vi "Visualize_MutationHistory_Path.vi"(8 "error in (no error)":errorcluster, 10 "LVClass library Path":path, 11 "class reference":refnum<vi>) -> (0 "error out":errorcluster)   [LabVIEW 2019, in "BlueSerializationScripts.lvlib"]
uses:
  BlueSerializationScripts.lvlib
  BlueUtilityScripts/BlueUtilityScripts.lvlib
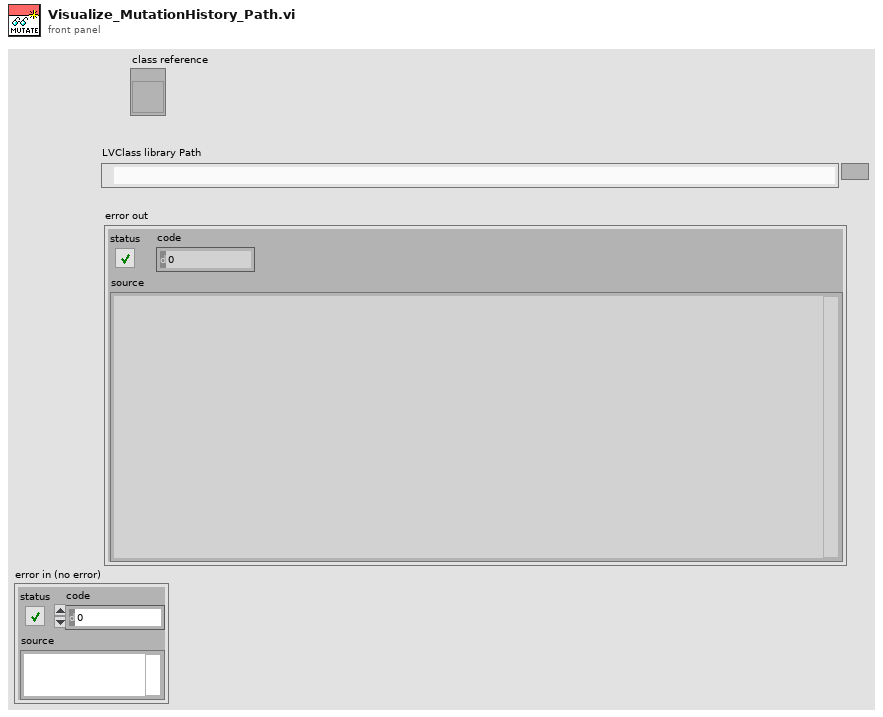
[diagram p1: front panel]
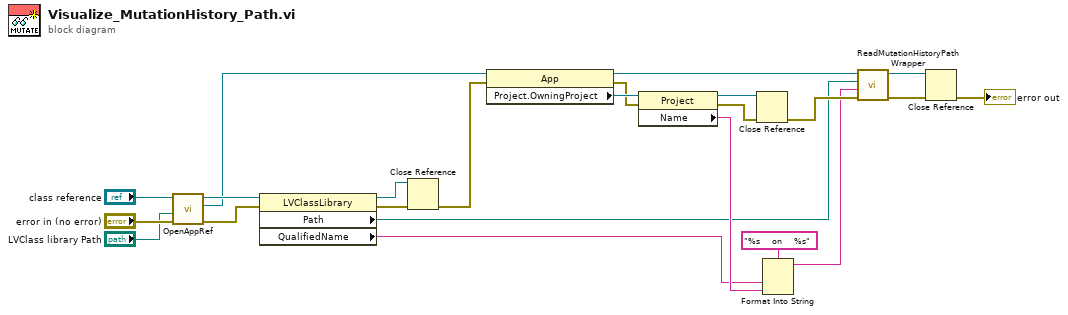
[diagram p0: block diagram]
diagram:
  n1 = call "OpenAppRef.vi"("error in (no error)"="error in (no error)", "LVClass library Path"="LVClass library Path", "class reference"="class reference") -> ("error out"=w17:errorcluster, "Application reference"=w14:refnum<vi>, "LVClass Reference"=w18:refnum<vi>)  [unwired: 6 in]
  n2 = property class="LVClassLibrary"(reference=w18, error in=w17) -> (reference out=w16:refnum<vi>, error out=w15:errorcluster, "Path"=w3:path, "QualifiedName"=w4:string)
  n3 = Close Reference(reference=w16, error in (no error)=w15) -> (error out=w6:errorcluster)
  n4 = property class="App"(reference=w14, error in=w6) -> (reference out=w10:refnum<vi>, error out=w9:errorcluster, "Project.OwningProject"=w13:refnum<vi>)
  n5 = property class="Project"(reference=w13, error in=w9) -> (reference out=w8:refnum<vi>, error out=w7:errorcluster, "Name"=w11:string)
  n6 = Close Reference(reference=w8, error in (no error)=w7) -> (error out=w5:errorcluster)
  n7 = Format Into String(format string="%s    on    %s", w4, w11) -> (resulting string=w2:string)  [unwired: 2 in, 1 out]
  n8 = call "ReadMutationHistoryPathWrapper.vi"("error in (no error)"=w5, "Name"=w2, "LVClass path"=w3, "Application"=w10) -> ("error out"=w1:errorcluster, "Application"=w19:refnum<vi>)  [unwired: 6 in]
  n9 = Close Reference(reference=w19, error in (no error)=w1) -> (error out=→"error out":errorcluster)
